vi "Apply Transformations.vi"(8 "error in (no error)":errorcluster, 11 "Tool Rectangle in":refnum<class "Tool Rectangle.lvclass">) -> (0 "error out":errorcluster, 3 "Tool Rectangle out":refnum<class "Tool Rectangle.lvclass">)   [LabVIEW 2019, in "Tool Rectangle.lvclass"]
uses:
  Tool Rectangle.lvclass
  Parse/Rectangle/Rectangle.lvclass/Rectangle.ctl
  Parse/PathCommands/Point.ctl
  Parse/Transform/Transform.lvclass/Transform.ctl
  Parse/Rectangle/Read Transforms.vi
  Parse/Rectangle/Read Width.vi
  Parse/Rectangle/Read X.vi
  Parse/Rectangle/Read Height.vi
  Parse/Rectangle/Read Y.vi
  Parse/Transform/Transform.lvclass
  <vilib>/Analysis/baseanly.llb/Real A x B.vi
  Parse/PathCommands/PathCommands.lvclass
  <vilib>/Analysis/NI_AALBase.lvlib
  Parse/Rectangle/Rectangle.lvclass
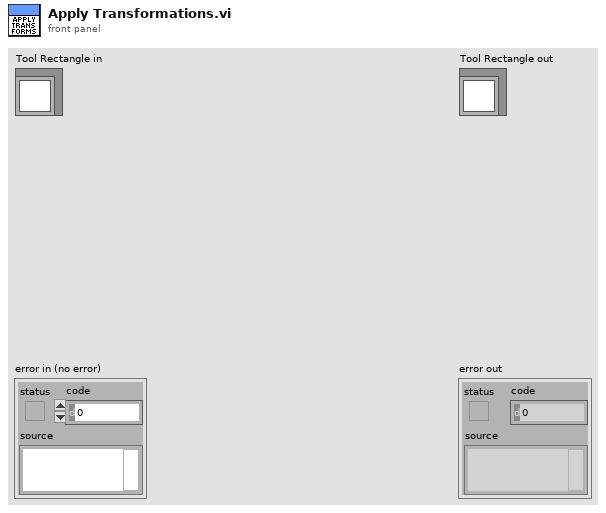
[diagram p1: front panel]
types:
  T1 = typedef "PathCommands.lvclass/Point.ctl" = cluster{"X":dbl, "Y":dbl}
  T2 = typedef "NI_Matrix.lvlib/RealMatrix.ctl" = dbl[][]
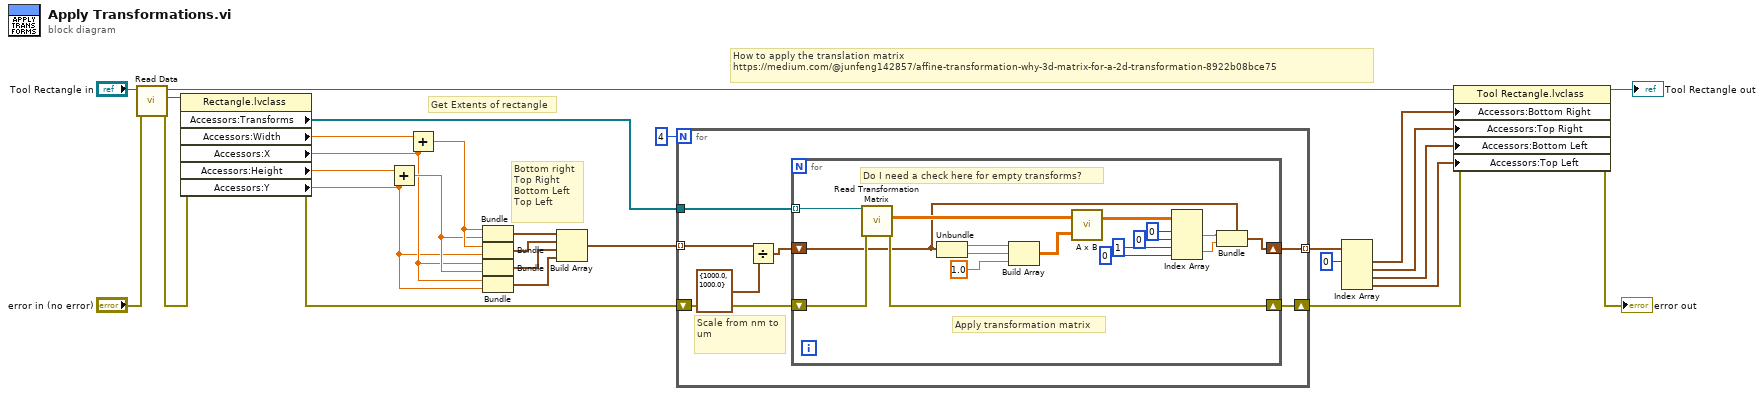
[diagram p0: block diagram]
diagram:
  # "Get Extents of rectangle"
  # "Bottom right\nTop Right\nBottom Left\nTop Left"
  # "How to apply the translation matrix\nhttps://medium.com/@junfeng142857/affine-transformation-why-3d-matrix-for-a-2d-transformation-8922b08bce75"
  n1 = call-dynamic "Read Data.vi"("error in (no error)"="error in (no error)", "Tool Rectangle in"="Tool Rectangle in") -> ("error out"=w24:errorcluster, "Rectangle.lvclass"=w27:refnum<class "Rectangle.lvclass">, "Tool Rectangle out"=w13:refnum<class "Tool Rectangle.lvclass">)  [unwired: 7 in]
  n2 = property class="Rectangle.lvclass"(reference=w27, error in=w24) -> (error out=w25:errorcluster, "Accessors:Transforms"=w26:refnum<class "Transform.lvclass">[], "Accessors:Width"=w23:dbl, "Accessors:X"=w6:dbl, "Accessors:Height"=w22:dbl, "Accessors:Y"=w5:dbl)  [unwired: 1 out]
  n3 = Add(x=w22, y=w5) -> (x+y=w20:dbl)
  n4 = Add(x=w23, y=w6) -> (x+y=w21:dbl)
  n5 = Bundle(w21, w20) -> (w18:cluster{dbl, dbl})  [unwired: 1 in]
  n6 = Bundle(w21, "Accessors:Y"=w5) -> (w15:cluster{dbl, "Accessors:Y":dbl})  [unwired: 1 in]
  n7 = Bundle("Accessors:X"=w6, w20) -> (w17:cluster{"Accessors:X":dbl, dbl})  [unwired: 1 in]
  n8 = Bundle("Accessors:X"=w6, "Accessors:Y"=w5) -> (w16:cluster{"Accessors:X":dbl, "Accessors:Y":dbl})  [unwired: 1 in]
  n9 = Build Array(w18, w15, w17, w16) -> (w7:cluster{"Accessors:X":dbl, "Accessors:Y":dbl}[])
  n10 = for {
    N: 4 -> [_]
    tunnel: w26 -> [w35]
    shift-right: [w31] -> w3
    shift-left: w25 -> [w34]
    tunnel: w7 -> [w30] mode=indexing
    tunnel: [w29] -> w4 mode=indexing
    # "Scale from nm to um"
    n11 = Divide(x=w30, y=T1 {"X"=1000.0, "Y"=1000.0} ("Point")) -> (x/y=w32:T1)
    n12 = for {
      tunnel: w35 -> [w52] mode=indexing
      shift-right: [w36] -> w29
      shift-left: w32 -> [w48]
      shift-right: [w49] -> w31
      shift-left: w34 -> [w50]
      # "Apply transformation matrix"
      # "Do I need a check here for empty transforms?"
      n13 = call "Read Transformation Matrix.vi"("error in (no error)"=w50, "Transform in"=w52) -> ("error out"=w49:errorcluster, "Real Matrix"=w51:T2)  [unwired: 7 in, 1 out]
      n14 = Unbundle(w48) -> ("X"=w47:dbl, "Y"=w46:dbl)
      n15 = Build Array(w47, w46, 1.0) -> (w37:T2)
      n16 = call-poly <vilib>:"A x B.vi"("B"=w37, "A"=w51) -> ("A x B"=w45:T2)  [unwired: 1 out]
      n17 = Index Array(array=w45, index (row) #1=0 ("index (row)"), index (col) #1=0 ("index (col)"), index (row) #2=1 ("index (row)"), index (col) #2=0 ("index (col)")) -> (element #1=w41:dbl, element #2=w40:dbl)
      n18 = Bundle(cluster=w48, "X"=w41, "Y"=w40) -> (w36:T1)
    }
  }
  n19 = Index Array(array=w4, index #1=0 ("index")) -> (element #1=w11:T1, element #2=w10:T1, element #3=w9:T1, element #4=w8:T1)  [unwired: 3 in]
  n20 = property class="Tool Rectangle.lvclass"(reference=w13, error in=w3, "Accessors:Bottom Right"=w11, "Accessors:Top Right"=w10, "Accessors:Bottom Left"=w9, "Accessors:Top Left"=w8) -> (reference out=→"Tool Rectangle out":refnum<class "Tool Rectangle.lvclass">, error out=→"error out":errorcluster)
